vi "TPNT_GetTPfromDevice.vi"(6 "attempts":i32, 8 "error in (no error)":errorcluster, 9 "device interface":string, 10 "device name":string, 11 "testpoint name":string) -> (0 "error out":errorcluster, 2 "value out":string)   [LabVIEW 2016]
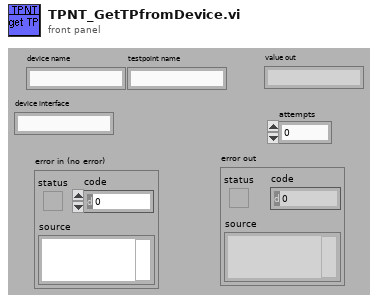
[diagram p1: front panel]
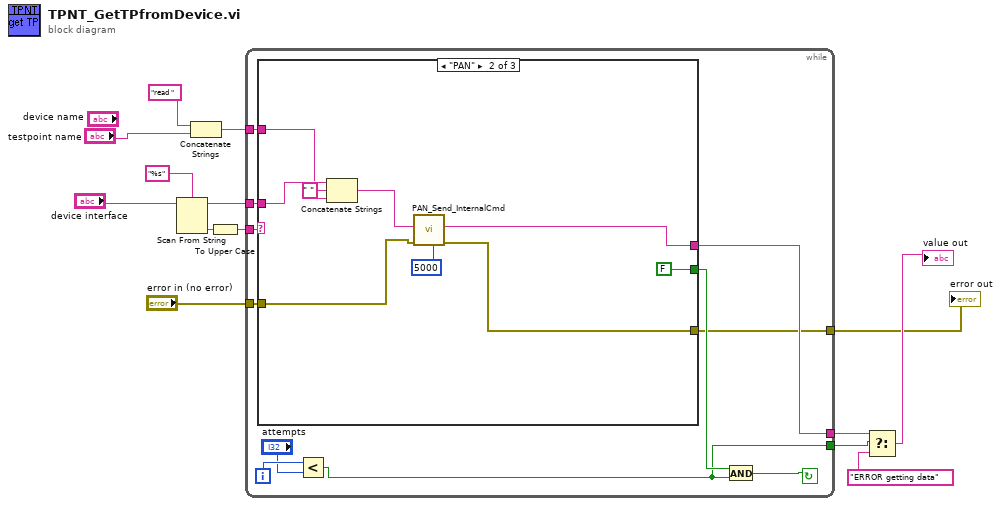
[diagram p0: block diagram]
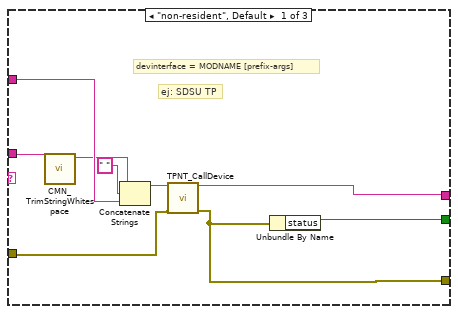
[diagram p2: hidden frame]
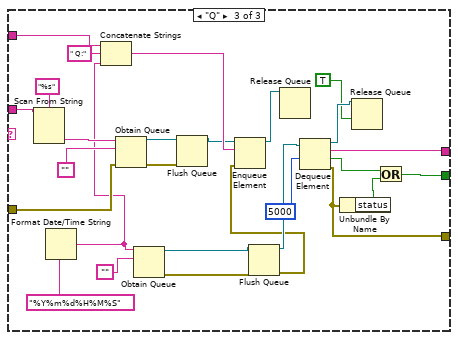
[diagram p3: hidden frame]
diagram:
  n1 = Scan From String(format string="%s", input string="device interface") -> (remaining string=w10:string, output 1=w12:string)  [unwired: 2 in, 3 out]
  n2 = Concatenate Strings("read " ("string"), "testpoint name") -> (w1:string)
  n3 = To Upper Case(1:w12) -> (0:w11:string)
  n4 = while {
    tunnel: w11 -> [w25]
    tunnel: w10 -> [w24]
    tunnel: [w16] -> w9
    tunnel: [w19] -> w7
    tunnel: "error in (no error)" -> [w18]
    tunnel: [w17] -> w4
    tunnel: w1 -> [w15]
    i -> [w23]
    stop <- w20 continue-if-true
    n5 = case shown="\"PAN\"" w25 {
      tunnel: w24 -> [w27 w43 w70]
      tunnel: [w28 FALSE ("status") w64] -> w21
      tunnel: [w30 w40 w63] -> w19
      tunnel: w18 -> [w31 w38 w61]
      tunnel: [w29 w37 w60] -> w17
      tunnel: w15 -> [w33 w41 w57]
      frame "non-resident", Default {
        # "ej: SDSU TP"
        # "devinterface = MODNAME [prefix-args]"
        n6 = call "CMN_TrimStringWhitespace.vi"("string"=w27) -> ("trimmed string"=w26:string)  [unwired: 1 in, 8 out]
        n7 = Concatenate Strings(w26, " " ("string"), w33) -> (w32:string)
        n8 = call "TPNT_CallDevice.vi"("CmdStringIn"=w32, "error in (no error)"=w31) -> ("ImmedReplyString"=w30:string, "error out"=w29:errorcluster)  [unwired: 12 out]
        n9 = Unbundle By Name(w29) -> ("status"=w28:bool)
      }
      frame "PAN" {
        n10 = Concatenate Strings(w43, " " ("string"), w41) -> (w42:string)
        n11 = call "PAN_Send_InternalCmd.vi"("timeout in ms (-1)"=5000, "error in (no error)"=w38, "command"=w42) -> ("error out"=w37:errorcluster, "response"=w40:string)  [unwired: 2 in, 5 out]
      }
      frame "Q" {
        n12 = Scan From String(format string="%s", input string=w70) -> (output 1=w59:string)  [unwired: 2 in, 4 out]
        n13 = Format Date/Time String(time format string (%c)="%Y%m%d%H%M%S") -> (date/time string=w53:string)  [unwired: 2 out]
        n14 = Concatenate Strings(w57, " Q:" ("string"), w53) -> (w55:string)
        n15 = Obtain Queue(name (unnamed)=w59, element data type="", error in (no error)=w61) -> (queue out=w47:refnum<queue>, error out=w45:errorcluster)  [unwired: 2 in, 1 out]
        n16 = Obtain Queue(name (unnamed)=w53, element data type="") -> (queue out=w51:refnum<queue>, error out=w50:errorcluster)  [unwired: 3 in, 1 out]
        n17 = Flush Queue(queue=w47, error in (no error)=w45) -> (queue out=w46:refnum<queue>)  [unwired: 2 out]
        n18 = Flush Queue(queue=w51, error in (no error)=w50) -> (queue out=w49:refnum<queue>, error out=w48:errorcluster)  [unwired: 1 out]
        n19 = Enqueue Element(queue=w46, element=w55, error in (no error)=w48) -> (queue out=w54:refnum<queue>)  [unwired: 3 out]
        n20 = Release Queue(queue=w54) -> ()  [unwired: 1 in, 4 out]
        n21 = Dequeue Element(queue=w49, timeout in ms (-1)=5000) -> (queue out=w62:refnum<queue>, element=w63:string, timed out?=w66:bool, error out=w60:errorcluster)  [unwired: 1 in]
        n22 = Unbundle By Name(w60) -> ("status"=w65:bool)
        n23 = Release Queue(queue=w62, force destroy? (F)=TRUE) -> ()  [unwired: 1 in, 3 out]
        n24 = Or(x=w66, y=w65) -> (x .or. y?=w64:bool)
      }
    }
    n25 = Less?(x=w23, y="attempts") -> (x < y?=w16:bool)
    n26 = And(x=w21, y=w16) -> (x .and. y?=w20:bool)
  }
  "error out" <- w4
  n27 = Select(t=w7, s=w9, f="ERROR getting data") -> (s? t:f=→"value out":string)
